vi "to DBL.vi"(8 "error in":errorcluster, 11 "bytes":u8[](array[numeric]) format="%b") -> (0 "error out":errorcluster, 3 "DBL":dbl)   [LabVIEW 2020, in "wamplv.lvlib" / "MessagePack.lvclass"]
uses:
  MessagePack.lvclass
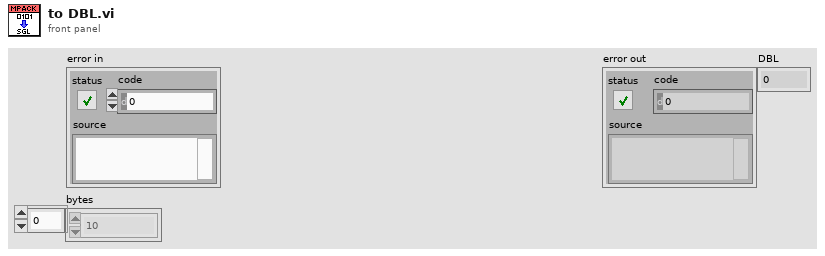
[diagram p1: front panel]
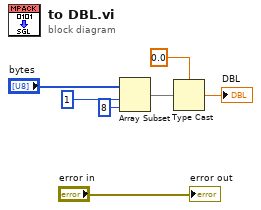
[diagram p0: block diagram]
diagram:
  n1 = Array Subset(array="bytes", index=1, length=8) -> (w3:u8[])
  n2 = Type Cast(type=0.0 ("DBL"), x=w3) -> (*(type *) &x=→"DBL":dbl)
  "error out" <- "error in"
